vi "Calculate Derived Stroker Analog Variables.vi"(6 "Lower Tension Sub Data":dbl[](array[numeric]), 7 "Selected Tool":T1, 8 "Upper Tension Sub Data":dbl[](array[numeric]), 9 "Solenoid Analog Data":dbl[](array[numeric]), 10 "Pressure 2 Analog Data":dbl[](array[numeric]), 11 "Pressure 1 Analog Data":dbl[](array[numeric])) -> (2 "Stroker Data Out":dbl[](array[numeric]))   [LabVIEW 2011]
uses:
  List of tools.ctl
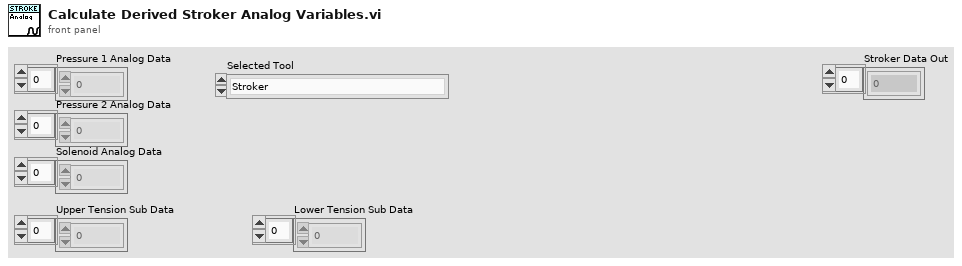
[diagram p1: front panel]
types:
  T1 = typedef "List of tools.ctl" = enum16{"Stroker", "Driller", "Tractor"}
  T2 = typedef "Options  All pages and custom.ctl" = cluster{"P 1 (App)":T3, "P 2":T4, "P 3":T5, "P 4":T8, "P 5":T13, "P 6 (Err)":T14, "P 7 (Expert)":T15, "P 8 (Depth)":T17, "C 1":T18, "C 2":T19}
  T3 = typedef "Options Page 1 (App).ctl" = cluster{"Result files":path, "PCP Interface":string, "Tractor/Stroker Interface":string, "Tractor Interface":string, "Modem Status Interface":string, "Audible Alarm":bool, "Force alarm on Technical":bool, "Force alarm on HH":bool, "Force alarm on LL":bool, "Force alarm on H":bool, "Force alarm on L":bool}
  T4 = typedef "Options Page 2.ctl" = cluster{"Solenoid & Relay latching time":u16, "Tractor relay 1":dbl, "Tractor relay 2":dbl, "Tractor Solenoid limit":dbl}
  T5 = typedef "Options Page 3.ctl" = cluster{"Min resistance":dbl, "Max resistance":dbl, "Head voltage range":T6, "Max voltage jump":dbl, "Maximum resistance change":dbl, "Start Telemetry Voltage":dbl, "Start Telemetry Timeout":dbl, "Start Motor Voltage":dbl, "Stop Motor Voltage":dbl, "Pass Mode Warning Voltage":dbl, "Relay Switch Voltage":dbl, "Relay Status Loss Voltage":dbl, "Samples to average":i32, "PSU type DO NOT USE":T7, "Magna OVP":dbl, "Magna Current Limit":dbl}
  T6 = typedef "PCP type List.ctl" = enum16{"0 - 350V", "0 - 450V", "0 - 600V"}
  T7 = typedef "PSU Type.ctl" = enum16{"Unipower", "Magna 8.3A", "Magna 12A", "None"}
  T8 = typedef "Options Page 4.ctl" = cluster{"Solenoid & Relay latching time":u16, "Stroker relay 1":dbl, "Stroker Relay 2":dbl, "Stroker Solenoid limit":dbl, "Force det.":T9, "Stroke force lim.":dbl, "Anchor Enabled Pressure":dbl, "Tacometer puls":dbl, "Default anchor behavior":T10, "Default stroker behavior":T11, "Default stroker force limit (tonne)":dbl, "Slips Size":T12}
  T9 = typedef "Stroke force selector.ctl" = enum16{"Stroke in = node 1", "Strok out = node 1"}
  T10 = typedef "Default anchor behavior.ctl" = enum16{"Do nothing", "Set Anchor", "Release Anchor"}
  T11 = typedef "Default stroker behavior.ctl" = enum16{"Do nothing", "Stop", "Go Out", "Go In"}
  T12 = typedef "Slips Type Radio.ctl" = enum32{"No Selection", "338 MRS", "3,9 MRS"}
  T13 = typedef "Options Page 5.ctl" = cluster{"Solenoid & Relay latching time":u16, "Driller relay 1":dbl, "Driller Relay 2":dbl, "Driller  Solenoid limit":dbl}
  T14 = typedef "Options Page 6 (Err).ctl" = cluster{"Error and event files":path}
  T15 = typedef "Options Page 7 (Expert).ctl" = cluster{"Show Debug":bool, "Log debug messages":bool, "Additional debug messages":bool, "Start Beagle with Simulator data":bool, "Workshop mode":bool, "Modem baud":u16, "enumCANCOM":bool, "Modem sim":T16, "Telemetry Timeout Disable":i32, "Buffer size":i32, "Upd regular data":bool, "Cable comp":cluster{"VMOD1 Voltage(V)":dbl, "VMOD2 Voltage(V)":dbl}}
  T16 = typedef "Modem simulation setup.ctl" = cluster{"Modem dealay sim":bool, "Sim baud Tx":u16, "Bit Error fraction Tx":dbl, "Sim baud Rx":u16, "Bit Error fraction Rx":dbl}
  T17 = typedef "Options Page 8 (Depth).ctl" = cluster{"Winch Spool Circumference":dbl, "Winch Pulses per Revolution":dbl, "Current Depth":dbl}
  T18 = typedef "Options Custom 1.ctl" = cluster{"Depth Updated":bool, "Depth Offset":dbl}
  T19 = typedef "Options Custom 2.ctl" = cluster{"Placeholder":bool}
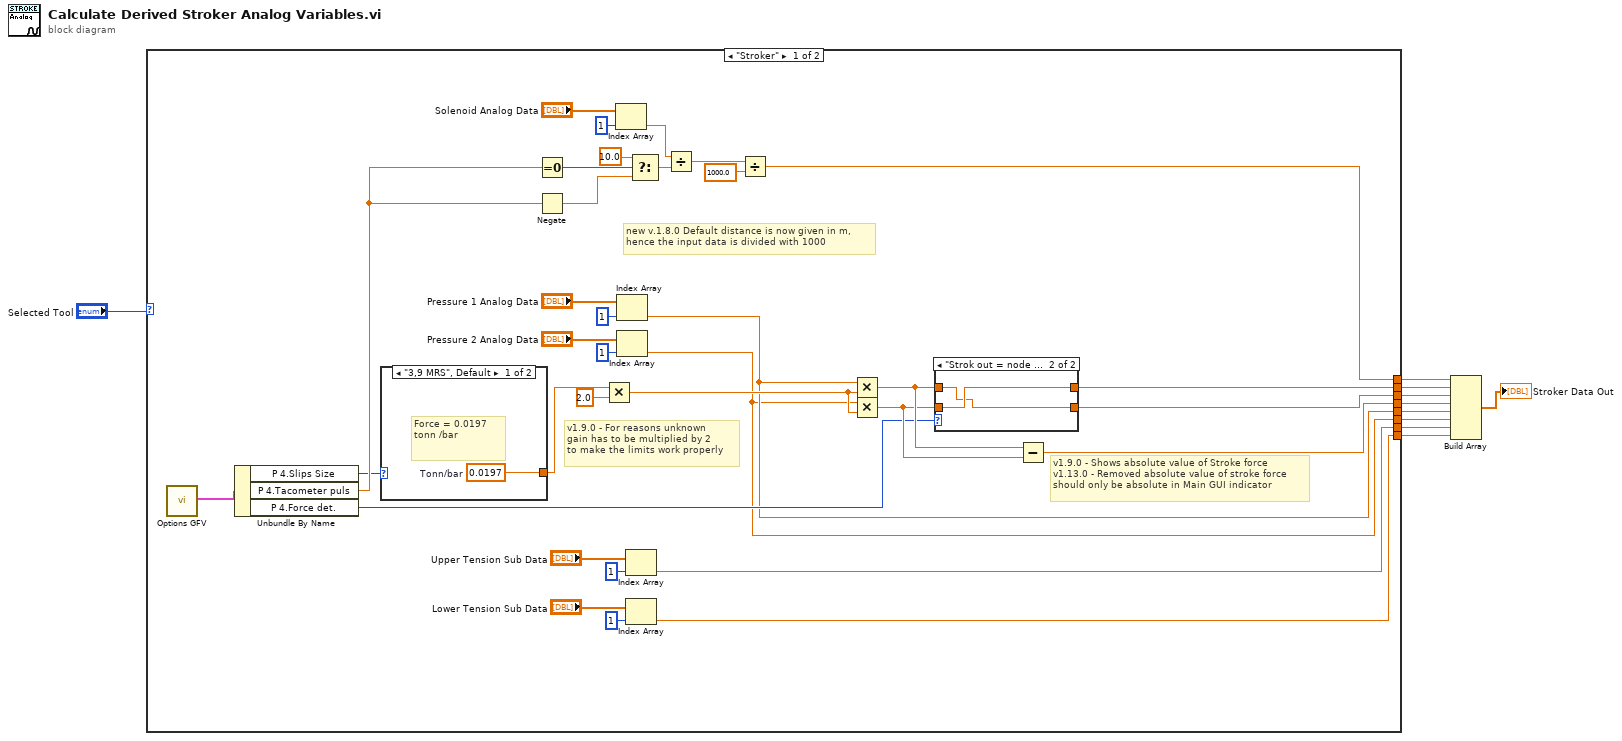
[diagram p0: block diagram]
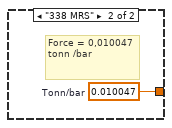
[diagram p2: hidden frame]
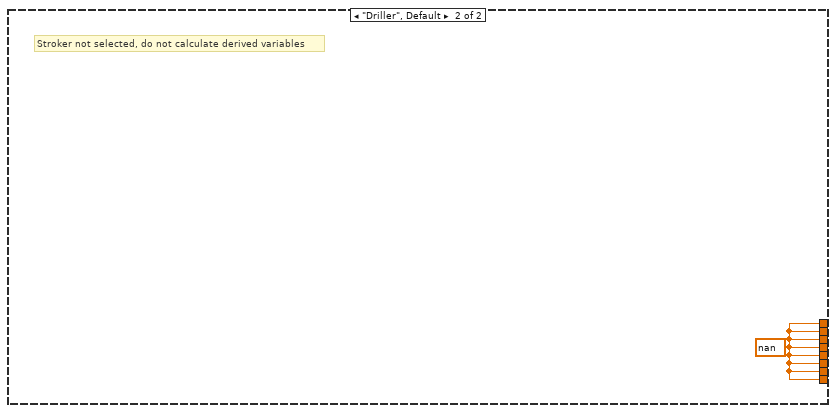
[diagram p4: hidden frame]
diagram:
  n1 = case shown="\"Stroker\"" "Selected Tool" {
    tunnel: [w44 w51] -> w10
    tunnel: [w43 w51] -> w9
    tunnel: [w13 w51] -> w8
    tunnel: [w22 w51] -> w6
    tunnel: [w21 w51] -> w4
    tunnel: [w20 w51] -> w3
    tunnel: [w15 w51] -> w2
    tunnel: [w14 w51] -> w1
    frame "Stroker" {
      # "new v.1.8.0 Default distance is now given in m, \nhence the input data is divided with 1000"
      # "v1.9.0 - For reasons unknown \ngain has to be multiplied by 2\nto make the limits work properly"
      # "v1.9.0 - Shows absolute value of Stroke force\nv1.13.0 - Removed absolute value of stroke force\nshould only be absolute in Main GUI indicator"
      n2 = call "Options GFV.vi"() -> ("Options"=w32:T2)  [unwired: 17 in, 2 out]
      n3 = Unbundle By Name(w32) -> ("P 4.Slips Size"=w12:T12, "P 4.Tacometer puls"=w24:dbl, "P 4.Force det."=w31:T9)
      n4 = case shown="\"3,9 MRS\", Default" w12 {
        tunnel: [w45 w46] -> w11
        frame "3,9 MRS", Default {
          w45 = 0.0197  # Tonn/bar
          # "Force = 0.0197 tonn /bar"
        }
        frame "338 MRS" {
          w46 = 0.010047  # Tonn/bar
          # "Force = 0,010047 tonn /bar"
        }
      }
      n5 = Equal To 0?(x=w24) -> (x = 0?=w27:bool)
      n6 = Negate(x=w24) -> (-x=w25:dbl)
      n7 = Multiply(x=w11, y=2.0) -> (x*y=w33:dbl)
      n8 = Index Array(array="Solenoid Analog Data", index=1) -> (element=w23:dbl)
      n9 = Index Array(array="Pressure 1 Analog Data", index=1) -> (element=w21:dbl)
      n10 = Index Array(array="Pressure 2 Analog Data", index=1) -> (element=w20:dbl)
      n11 = Index Array(array="Upper Tension Sub Data", index=1) -> (element=w15:dbl)
      n12 = Index Array(array="Lower Tension Sub Data", index=1) -> (element=w14:dbl)
      n13 = Select(t=10.0, s=w27, f=w25) -> (s? t:f=w30:dbl)
      n14 = Divide(x=w23, y=w30) -> (x/y=w29:dbl)
      n15 = Divide(x=w29, y=1000.0) -> (x/y=w22:dbl)
      n16 = Multiply(x=w21, y=w33) -> (x*y=w42:dbl)
      n17 = Multiply(x=w20, y=w33) -> (x*y=w41:dbl)
      n18 = case shown="\"Strok out = node 1\"" w31 {
        tunnel: w42 -> [w48 w49]
        tunnel: w41 -> [w47 w50]
        tunnel: [w48 w50] -> w44
        tunnel: [w47 w49] -> w43
        frame "Stroke in = node 1", Default {
        }
        frame "Strok out = node 1" {
        }
      }
      n19 = Subtract(x=w42, y=w41) -> (x-y=w13:dbl)
    }
    frame "Driller", Default {
      w51 = nan
      # "Stroker not selected, do not calculate derived variables"
    }
  }
  n20 = Build Array(w6, w10, w9, w8, w4, w3, w2, w1) -> (→"Stroker Data Out":dbl[])
